vi "AI algorithm (SubVI).vi"(8 "Q option":i32, 9 "Jump?":bool, 10 "y":i32, 11 "x":i32) -> (2 "Next Action":i32, 3 "Q":dbl[][](array[numeric]))   [LabVIEW 2013]
doc: "Uses reinforcement learning to learn from failure and generates the strategy for the next action. This vi is developed for the flappy bird project."
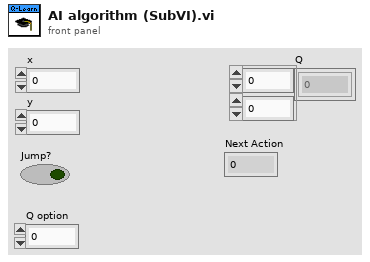
[diagram p1: front panel]
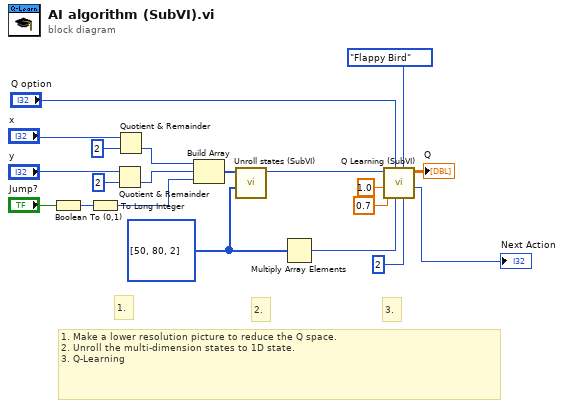
[diagram p0: block diagram]
diagram:
  w14 = i32[] [50, 80, 2] ("# each state")
  # "3."
  # "2."
  # "1."
  # "1. Make a lower resolution picture to reduce the Q space.\n2. Unroll the multi-dimension states to 1D state.\n3. Q-Learning"
  n1 = Boolean To (0,1)(Boolean="Jump?") -> (0, 1=w4:i16)
  n2 = To Long Integer(number=w4) -> (32bit integer=w20:i32)
  n3 = Quotient & Remainder(x="y", y=2) -> (floor(x/y)=w11:i32)  [unwired: 1 out]
  n4 = Quotient & Remainder(x="x", y=2) -> (floor(x/y)=w2:i32)  [unwired: 1 out]
  n5 = Build Array(w2, w11, w20) -> (w19:i32[])
  n6 = call "Unroll states (SubVI).vi"("size of each state"=w14, "State array"=w19) -> ("Unrolled state"=w15:i32)  [unwired: 9 in]
  n7 = Multiply Array Elements(1:w14) -> (0:w13:i32)
  n8 = call "Q Learning (SubVI).vi"("# action"=2, "Mode"=enum16{"Algorithm test", "Flappy Bird"}."Flappy Bird", "# state"=w13, "Q option"="Q option", "alpha"=0.7, "Gamma"=1.0, "State"=w15) -> ("Next Action"=→"Next Action":i32, "Q"=→"Q":dbl[][])  [unwired: 3 in]
